vi "ET3500 - Write Program.vi"(5 "Simulate":bool caption="Simulate ET3500", 8 "Error In":errorcluster, 9 "MCListBox FHS Setup":refnum<vi>, 10 "WPS Details Setup":T3={"WPS/Ref"="", "Rev"="", "Hold Temperature"="80", "WPS Details Temperature Units"="DegC", "Hold Time (HH:MM)"="01:00", "Inactive"=FALSE} caption="WPS Details", 11 "VISA resource name RS232":string="visa://192.168.1.50/ASRL1::INSTR") -> (0 "ET3500":errorcluster, 1 "Final Target Temperture":i32, 2 "Duplicate Index":bool, 3 "Valid":bool, 4 "ET3500 Segment Table":i32[][](array[numeric])=[[1, 50, 400, 1], [2, 30, 500, 1], [3, 15, 600, 1], [4, 0, 0, 3], [5, 0, 0, 0]], 6 "Seq-Seg Info":T1)   [LabVIEW 2013]
uses:
  Controls/Combo Box.ctl
  Controls/ET3500 Enum.ctl
  Controls/ET3500 Programmer Enum.ctl
  Controls/ET3500 Segment Enum.ctl
panel:
  in  "Rev2":string="MyWPS55" caption="Rev"
  in  "Extra WPS":string="MyWPS55" caption="WPS"
  out "Old":i32[][](array[numeric])=[[1, 30, 300, 1], [2, 70, 600, 1], [0, 0, 0, 3], [5, 50, 400, 1], [0, 0, 0, 0]]
  out "Segment.Holdback":i32[](array[numeric])
  in  "ProgramNumber":i32=33
  out "num of rows\n(including blank row)":i32=4
  out "Main Hold Time (min)":dbl=270.0
  in  "MCListBox FHS Setup":i32(listbox)=-1 caption="Furnance Heating Sequence"
  # "visa://192.168.1.50/ASRL1::INSTR"
  # "Extra Fields used in SETUP ONLY"
  # "Sequence#       Ramp Rate       Target Temp          Hold Time       SegType"
  # "0 - NA\n1 - Low\n2 - High"
  # "Seq Num        Ramp Rate       Target Temp            SegType"
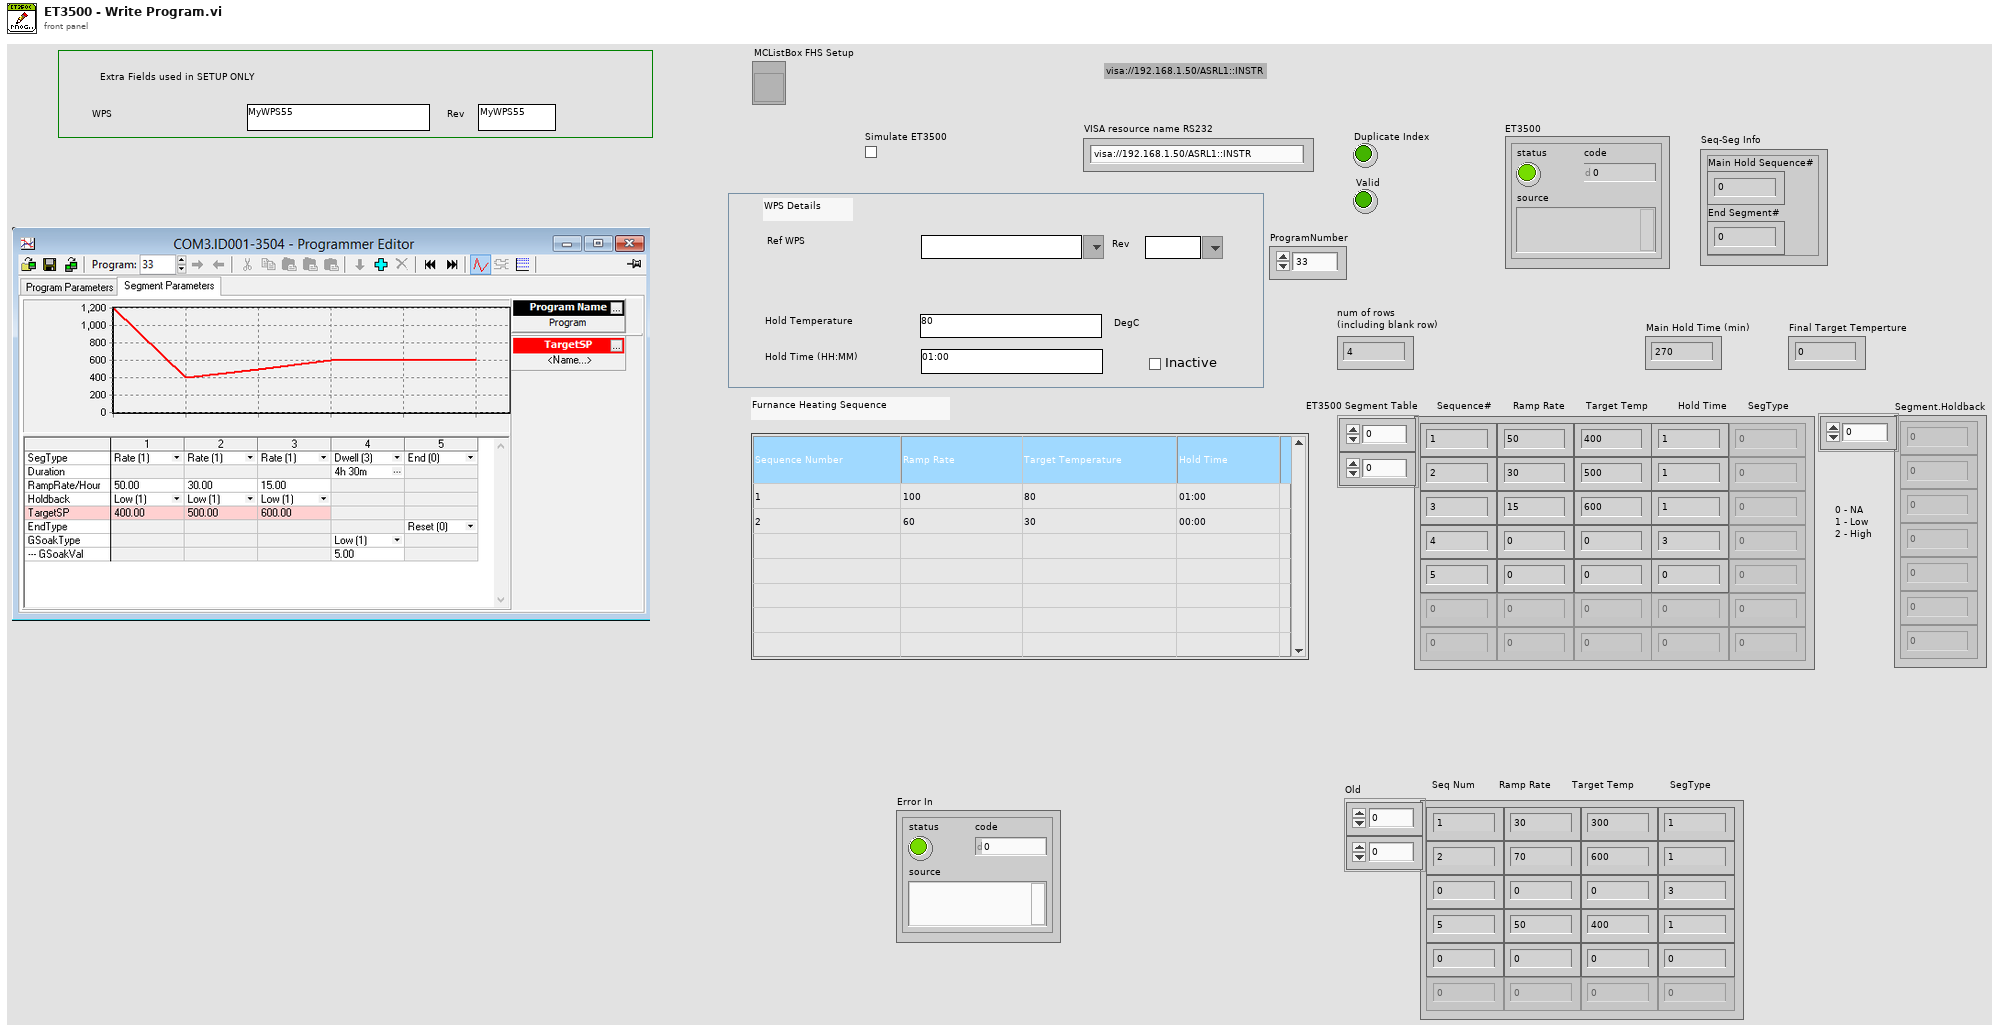
[diagram p1: front panel]
types:
  T1 = cluster{"Main Hold Sequence#":i32, "End Segment#":i32}
  T2 = typedef "Combo Box.ctl" = string
  T3 = cluster{"WPS/Ref":T2, "Rev":T2, "Hold Temperature":string, "WPS Details Temperature Units":string, "Hold Time (HH:MM)":string, "Inactive":bool}
  T4 = typedef "Enum - InteractiveMode-SubVIMode.ctl" = enum16{"Interactive", "subVI Mode"}
  T5 = typedef "ET3500 Enum.ctl" = enum16{"Programmer1", "Segment1", "Segment2", "Segment3", "Segment4", "Segment5", "Segment6", "Segment7", "Segment8", "Segment9", "Segment10", "Segment11", "Segment12", "Segment13", "Segment14", "Segment15", "Segment16"}
  T6 = typedef "ET3500 Programmer Enum.ctl" = u16
  T7 = typedef "ET3500 Segment Enum.ctl" = u16
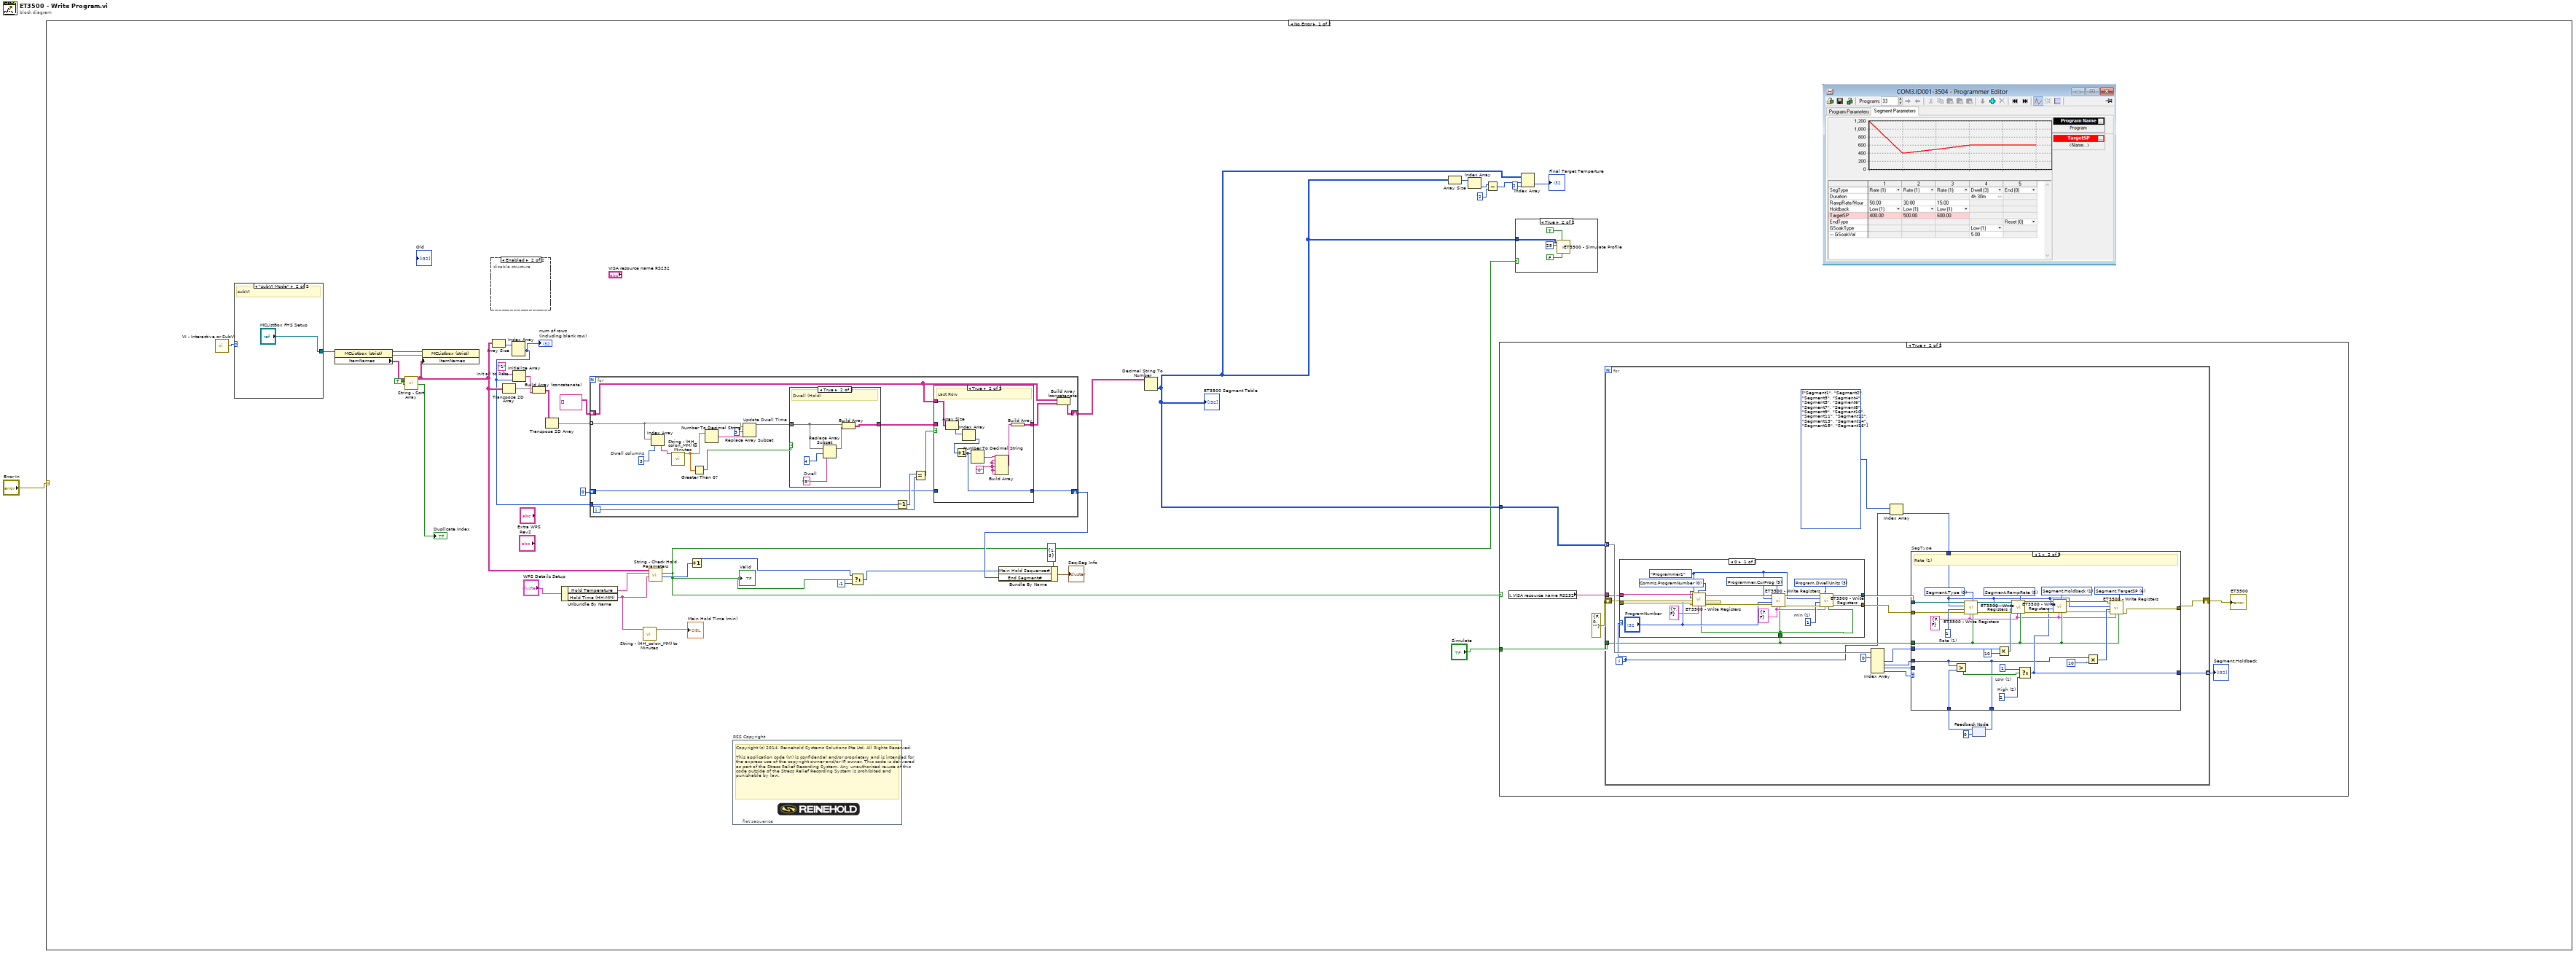
[diagram p0: block diagram]
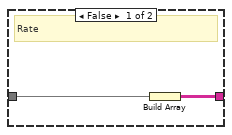
[diagram p3: hidden frame]
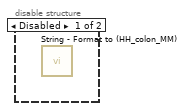
[diagram p4: hidden frame]
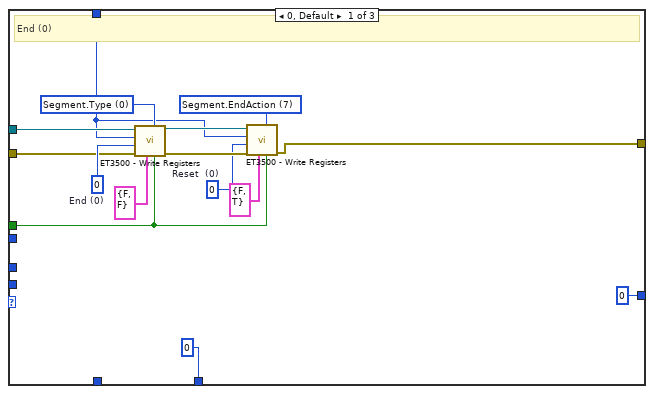
[diagram p8: hidden frame]
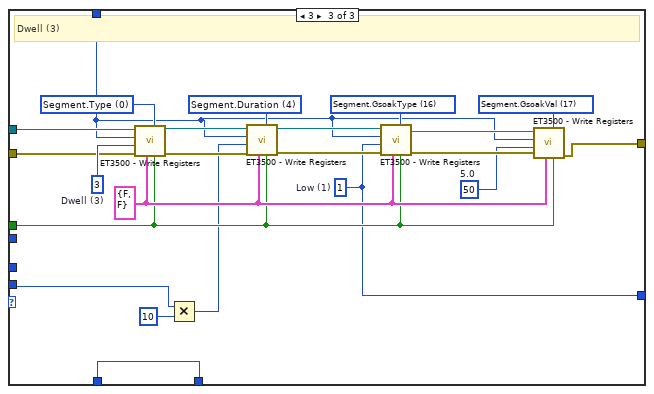
[diagram p9: hidden frame]
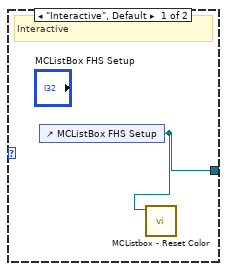
[diagram p10: hidden frame]
diagram:
  n1 = case shown="No Error" "Error In" {
    frame No Error {
      w12 = "1"  # Init all to Rate
      w11 = TRUE ("Check and Add Empty Row if Neccsary")
      n2 = call "VI - Interactive or SubVI.vi"() -> ("Mode"=w2:T4)  [unwired: 5 in]
      n3 = case shown="\"subVI Mode\"" w2 {
        tunnel: [w189 "MCListBox FHS Setup"] -> w34
        frame "Interactive", Default {
          # "Interactive"
          n4 = control-ref of="MCListBox FHS Setup"() -> (w189:refnum<vi>)
          n5 = call "MCListbox - Reset Color.vi"("MulticolumnListbox in"=w189) -> ()  [unwired: 10 in, 1 out]
        }
        frame "subVI Mode" {
          # "subVI"
        }
      }
      n6 = property class="MCListbox (strict)"(reference=w34) -> (reference out=w37:refnum<vi>, error out=w35:errorcluster, "ItemNames"=w36:string[][])  [unwired: 1 in]
      n7 = call "String - Sort Array.vi"("Force Running Numbers"=w11, "Check and Add Empty Row if Needed"=w11, "2D Array in"=w36) -> ("Duplicate Index"=→"Duplicate Index":bool, "2D Array out"=w19:string[][])  [unwired: 6 in, 1 out]
      n8 = property class="MCListbox (strict)"(reference=w37, error in=w35, "ItemNames"=w19) -> ()  [unwired: 2 out]
      n9 = disable-structure shown="Enabled" {
        frame Disabled {
          n10 = call "String - Format to (HH_colon_MM).vi"() -> ()  [unwired: 10 in, 2 out]
        }
        frame Enabled {
        }
      }
      n11 = Array Size(array=w19) -> (size(s)=w39:i32[])
      n12 = Transpose 2D Array(2D array=w19) -> (transposed array=w16:string[][])
      n13 = Index Array(array=w39) -> (element #1=w13:i32)  [unwired: 2 in, 1 out]
      "num of rows\n(including blank row)" <- w13
      n14 = Initialize Array(w12, w13) -> (w18:string[])
      n15 = Build Array (concatenate)(w16, w18) -> (w17:string[][])
      n16 = Transpose 2D Array(2D array=w17) -> (transposed array=w15:string[][])
      n17 = Unbundle By Name("WPS Details Setup") -> ("Hold Temperature"=w30:string, "Hold Time (HH:MM)"=w29:string)
      n18 = for {
        tunnel: w15 -> [w52] mode=indexing
        shift-right: [w53] -> w14
        shift-left: string[][] [] -> [w42]
        tunnel: w13 -> [w49]
        shift-right: [w41] -> w7
        shift-left: 0 -> [w40]
        i -> [w43]
        w54 = 3  # Dwell columns
        n19 = Index Array(array=w52, index=w54) -> (element=w57:string)
        n20 = call "String - (HH_colon_MM) to Minutes.vi"("Hold Time (HH:MM)"=w57) -> ("minutes"=w55:dbl)  [unwired: 10 in]
        n21 = Greater Than 0?(x=w55) -> (x > 0?=w56:bool)
        n22 = Number To Decimal String(number=w55) -> (decimal integer string=w51:string)  [unwired: 1 in]
        n23 = Replace Array Subset "Update Dwell Time"(array=w52, new element=w51, index=3) -> (w44:string[])
        n24 = case shown="True" w56 {
          tunnel: w44 -> [w68 w73]
          tunnel: [w69 w74] -> w46
          frame False {
            # "Rate"
            n25 = Build Array(w68) -> (w69:string[][])
          }
          frame True {
            w70 = "3"  # Dwell
            # "Dwell (Hold)"
            n26 = Replace Array Subset(array=w73, new element=w70, index=4) -> (w72:string[])
            n27 = Build Array(w73, w72) -> (w74:string[][])
          }
        }
        n28 = Decrement(x=w49) -> (x-1=w48:i32)
        n29 = Equal?(x=w48, y=w43) -> (x = y?=w47:bool)
        n30 = case shown="True" w47 {
          tunnel: w46 -> [w59 _]
          tunnel: [w59 w67] -> w45
          tunnel: w42 -> [_ w61]
          tunnel: [w58 w60] -> w41
          tunnel: w40 -> [w58 _]
          frame False {
          }
          frame True {
            w64 = "0" ("element")
            # "Last Row"
            n31 = Array Size(array=w61) -> (size(s)=w63:i32[])
            n32 = Index Array(array=w63) -> (element=w62:i32)  [unwired: 1 in]
            n33 = Increment(x=w62) -> (x+1=w60:i32)
            n34 = Number To Decimal String(number=w60) -> (decimal integer string=w66:string)  [unwired: 1 in]
            n35 = Build Array(w66, w64, w64, w64, w64, w64) -> (w65:string[])
            n36 = Build Array(w65) -> (w67:string[][])
          }
        }
        n37 = Build Array (concatenate)(w42, w45) -> (w53:string[][])
      }
      n38 = call "String - (HH_colon_MM) to Minutes.vi"("Hold Time (HH:MM)"=w29) -> ("minutes"=→"Main Hold Time (min)":dbl)  [unwired: 10 in]
      n39 = call "String - Check Hold Parameters.vi"("Master Data Hold Time (HH:MM)"=w29, "Master Data Hold Temperature"=w30, "2D Array in"=w19) -> ("index of Matched Hold Temperature"=w28:i32, "Found"=w6:bool)  [unwired: 6 in, 1 out]
      "Valid" <- w6
      n40 = Increment(x=w28) -> (x+1=w5:i32)
      n41 = flat-sequence "RSS Copyright" {
        frame #0 {
          # "Copyright (c) 2014, Reinehold Systems Solutions Pte Ltd. All Rights Reserved.\n\nThis application code (VI) is confidential and/or proprietary and is intended for the express use of the copyright owner and/or IP owner. This code is delivered as part of the Stress Relief Recording System. Any unauthorized re-use of this code outside of the Stress Relief Recording System is prohibited and punishable by law."
        }
      }
      n42 = Select(t=w5, s=w6, f=-1) -> (s? t:f=w3:i32)
      n43 = Bundle By Name(cluster=T1 {"Main Hold Sequence#"=1, "End Segment#"=5} ("Info"), "Main Hold Sequence#"=w3, "End Segment#"=w7) -> (→"Seq-Seg Info":T1)
      n44 = Decimal String To Number(string=w14) -> (number=w20:i32[][])  [unwired: 2 in, 1 out]
      "ET3500 Segment Table" <- w20
      n45 = Array Size(array=w20) -> (size(s)=w27:i32[])
      n46 = Index Array(array=w27) -> (element=w23:i32)  [unwired: 1 in]
      n47 = Subtract(x=w23, y=2 ("disabled index (col)")) -> (x-y=w26:i32)
      n48 = case shown="True" w6 {
        tunnel: w20 -> [_ w84]
        tunnel: "Simulate" -> [_ w80]
        frame False {
        }
        frame True {
          n49 = local read "VISA resource name RS232"() -> (w83:string)
          n50 = for {
            tunnel: w84 -> [w103] mode=indexing
            tunnel: w83 -> [w98]
            tunnel: w80 -> [w94]
            shift-right: [w99] -> w81
            shift-left: errorcluster {"status"=FALSE, "code"=0, "source"=""} ("error out") -> [w96]
            tunnel: [w90] -> w79 mode=indexing
            i -> [w92]
            w93 = T5[] [enum."Segment1", enum."Segment2", enum."Segment3", enum."Segment4", enum."Segment5", enum."Segment6", enum."Segment7", enum."Segment8", enum."Segment9", enum."Segment10", enum."Segment11", enum."Segment12", enum."Segment13", enum."Segment14", enum."Segment15", enum."Segment16"] items=["Programmer1", "Segment1", "Segment2", "Segment3", "Segment4", "Segment5", "Segment6", "Segment7", "Segment8", "Segment9", "Segment10", "Segment11", "Segment12", "Segment13", "Segment14", "Segment15", "Segment16"]
            n51 = case shown="0" w92 {
              tunnel: w98 -> [w116 w122]
              tunnel: [w112 w122] -> w97
              tunnel: w96 -> [w119 w121]
              tunnel: [w110 w121] -> w95
              tunnel: w94 -> [w104 _]
              frame 0 {
                w108 = 1  # min (1)
                w107 = T6 3 items=["Comms.ProgramNumber", "", "Program.RampUnits", "Program.DwellUnits", "", "", "", "", "", "Programmer.CurProg", "Programmer.CurSeg", "Programmer.ProgStatus", "", "", "", "", "", "Programmer.ProgTimeLeft", "Programmer.PVIn", "Programmer.SPIn", "", "Programmer.SegTimeLeft"] ("ET3500 Programmer Enum")
                w106 = T6 0 items=["Comms.ProgramNumber", "", "Program.RampUnits", "Program.DwellUnits", "", "", "", "", "", "Programmer.CurProg", "Programmer.CurSeg", "Programmer.ProgStatus", "", "", "", "", "", "Programmer.ProgTimeLeft", "Programmer.PVIn", "Programmer.SPIn", "", "Programmer.SegTimeLeft"] ("ET3500 Programmer Enum")
                w109 = ET3500_Enum."Programmer1" ("ET3500 Enum")
                w105 = cluster{"Init":bool, "Close":bool} {"Init"=FALSE, "Close"=FALSE} ("Option")
                w120 = T6 9 items=["Comms.ProgramNumber", "", "Program.RampUnits", "Program.DwellUnits", "", "", "", "", "", "Programmer.CurProg", "Programmer.CurSeg", "Programmer.ProgStatus", "", "", "", "", "", "Programmer.ProgTimeLeft", "Programmer.PVIn", "Programmer.SPIn", "", "Programmer.SegTimeLeft"] ("ET3500 Programmer Enum")
                n52 = call "ET3500 - Write Registers.vi"("Simulate"=w104, "Option"=cluster{"Init":bool, "Close":bool} {"Init"=TRUE, "Close"=FALSE}, "ET3500 Programmer Enum"=w106, "error in (no error)"=w119, "Process Variable  (0)"="ProgramNumber", "ET3500 Enum"=w109, "VISA resource name"=w116) -> ("error out"=w118:errorcluster, "VISA resource name out"=w117:refnum<visa-resource-name>)  [unwired: 3 in]
                n53 = call "ET3500 - Write Registers.vi"("Simulate"=w104, "Option"=w105, "ET3500 Programmer Enum"=w120, "error in (no error)"=w118, "Process Variable  (0)"="ProgramNumber", "ET3500 Enum"=w109, "VISA resource name"=w117) -> ("error out"=w111:errorcluster, "VISA resource name out"=w113:refnum<visa-resource-name>)  [unwired: 3 in]
                n54 = call "ET3500 - Write Registers.vi"("Simulate"=w104, "Option"=w105, "ET3500 Programmer Enum"=w107, "error in (no error)"=w111, "Process Variable  (0)"=w108, "ET3500 Enum"=w109, "VISA resource name"=w113) -> ("error out"=w110:errorcluster, "VISA resource name out"=w112:refnum<visa-resource-name>)  [unwired: 3 in]
              }
              frame 1, Default {
              }
            }
            n55 = Index Array(array=w103, index #1=0 ("index")) -> (element #2=w101:i32, element #3=w100:i32, element #4=w85:i32, element #5=w86:i32)  [unwired: 4 in, 1 out]
            n56 = Index Array(array=w93, index=w92) -> (element=w91:T5)
            n57 = feedback #1(0 ("String")) -> (w87:i32)
            n58 = case "SegType" shown="1" w86 {
              tunnel: w101 -> [_ w158 _]
              tunnel: w97 -> [w137 w165 w188]
              tunnel: w94 -> [w134 w148 w177]
              tunnel: w91 -> [w131 w154 w173]
              tunnel: w100 -> [_ w139 _]
              tunnel: [w127 w147 w171] -> w99
              tunnel: w95 -> [w126 w146 w182]
              tunnel: w85 -> [_ _ w166]
              tunnel: [0 ("Low (1)") w140 w168] -> w90
              tunnel: [0 ("String") w139 w167] -> w88
              tunnel: w87 -> [_ w138 w167]
              frame 0, Default {
                w129 = 0  # Reset  (0)
                w130 = T7 7 items=["Segment.Type", "Segment.Holdback", "", "", "Segment.Duration", "Segment.RampRate", "Segment.TargetSP", "Segment.EndAction", "", "", "", "", "", "", "", "", "Segment.GsoakType", "Segment.GsoakVal"] ("ET3500 Segment Enum")
                w136 = T7 0 items=["Segment.Type", "Segment.Holdback", "", "", "Segment.Duration", "Segment.RampRate", "Segment.TargetSP", "Segment.EndAction", "", "", "", "", "", "", "", "", "Segment.GsoakType", "Segment.GsoakVal"] ("ET3500 Segment Enum")
                w135 = 0  # End (0)
                # "End (0)"
                n59 = call "ET3500 - Write Registers.vi"("Simulate"=w134, "ET3500 Segment Enum"=w136, "Option"=cluster{"Init":bool, "Close":bool} {"Init"=FALSE, "Close"=FALSE}, "error in (no error)"=w126, "Process Variable  (0)"=w135, "ET3500 Enum"=w131, "VISA resource name"=w137) -> ("error out"=w133:errorcluster, "VISA resource name out"=w132:refnum<visa-resource-name>)  [unwired: 3 in]
                n60 = call "ET3500 - Write Registers.vi"("Simulate"=w134, "ET3500 Segment Enum"=w130, "Option"=cluster{"Init":bool, "Close":bool} {"Init"=FALSE, "Close"=TRUE}, "error in (no error)"=w133, "Process Variable  (0)"=w129, "ET3500 Enum"=w131, "VISA resource name"=w132) -> ("error out"=w127:errorcluster)  [unwired: 3 in, 1 out]
              }
              frame 1 {
                w141 = 2  # High (2)
                w142 = 1  # Low (1)
                w153 = T7 6 items=["Segment.Type", "Segment.Holdback", "", "", "Segment.Duration", "Segment.RampRate", "Segment.TargetSP", "Segment.EndAction", "", "", "", "", "", "", "", "", "Segment.GsoakType", "Segment.GsoakVal"] ("ET3500 Segment Enum")
                w145 = cluster{"Init":bool, "Close":bool} {"Init"=FALSE, "Close"=FALSE} ("Option")
                w155 = T7 1 items=["Segment.Type", "Segment.Holdback", "", "", "Segment.Duration", "Segment.RampRate", "Segment.TargetSP", "Segment.EndAction", "", "", "", "", "", "", "", "", "Segment.GsoakType", "Segment.GsoakVal"] ("ET3500 Segment Enum")
                w160 = T7 5 items=["Segment.Type", "Segment.Holdback", "", "", "Segment.Duration", "Segment.RampRate", "Segment.TargetSP", "Segment.EndAction", "", "", "", "", "", "", "", "", "Segment.GsoakType", "Segment.GsoakVal"] ("ET3500 Segment Enum")
                w164 = T7 0 items=["Segment.Type", "Segment.Holdback", "", "", "Segment.Duration", "Segment.RampRate", "Segment.TargetSP", "Segment.EndAction", "", "", "", "", "", "", "", "", "Segment.GsoakType", "Segment.GsoakVal"] ("ET3500 Segment Enum")
                w163 = 1  # Rate (1)
                # "Rate (1)"
                n61 = Greater?(x=w139, y=w138) -> (0:w143:bool)
                n62 = call "ET3500 - Write Registers.vi"("Simulate"=w148, "ET3500 Segment Enum"=w164, "Option"=w145, "error in (no error)"=w146, "Process Variable  (0)"=w163, "ET3500 Enum"=w154, "VISA resource name"=w165) -> ("error out"=w162:errorcluster, "VISA resource name out"=w161:refnum<visa-resource-name>)  [unwired: 3 in]
                n63 = Multiply(x=w158, y=10) -> (x*y=w157:i32)
                n64 = call "ET3500 - Write Registers.vi"("Simulate"=w148, "ET3500 Segment Enum"=w160, "Option"=w145, "error in (no error)"=w162, "Process Variable  (0)"=w157, "ET3500 Enum"=w154, "VISA resource name"=w161) -> ("error out"=w150:errorcluster, "VISA resource name out"=w156:refnum<visa-resource-name>)  [unwired: 3 in]
                n65 = Select(t=w142, s=w143, f=w141) -> (s? t:f=w140:i32)
                n66 = call "ET3500 - Write Registers.vi"("Simulate"=w148, "ET3500 Segment Enum"=w155, "Option"=w145, "error in (no error)"=w150, "Process Variable  (0)"=w140, "ET3500 Enum"=w154, "VISA resource name"=w156) -> ("error out"=w149:errorcluster, "VISA resource name out"=w144:refnum<visa-resource-name>)  [unwired: 3 in]
                n67 = Multiply(x=w139, y=10) -> (x*y=w151:i32)
                n68 = call "ET3500 - Write Registers.vi"("Simulate"=w148, "ET3500 Segment Enum"=w153, "Option"=w145, "error in (no error)"=w149, "Process Variable  (0)"=w151, "ET3500 Enum"=w154, "VISA resource name"=w144) -> ("error out"=w147:errorcluster)  [unwired: 3 in, 1 out]
              }
              frame 3 {
                w172 = T7 17 items=["Segment.Type", "Segment.Holdback", "", "", "Segment.Duration", "Segment.RampRate", "Segment.TargetSP", "Segment.EndAction", "", "", "", "", "", "", "", "", "Segment.GsoakType", "Segment.GsoakVal"] ("ET3500 Segment Enum")
                w176 = 50  # 5.0
                w168 = 1  # Low (1)
                w180 = T7 16 items=["Segment.Type", "Segment.Holdback", "", "", "Segment.Duration", "Segment.RampRate", "Segment.TargetSP", "Segment.EndAction", "", "", "", "", "", "", "", "", "Segment.GsoakType", "Segment.GsoakVal"] ("ET3500 Segment Enum")
                w178 = cluster{"Init":bool, "Close":bool} {"Init"=FALSE, "Close"=FALSE} ("Option")
                w183 = T7 4 items=["Segment.Type", "Segment.Holdback", "", "", "Segment.Duration", "Segment.RampRate", "Segment.TargetSP", "Segment.EndAction", "", "", "", "", "", "", "", "", "Segment.GsoakType", "Segment.GsoakVal"] ("ET3500 Segment Enum")
                w187 = T7 0 items=["Segment.Type", "Segment.Holdback", "", "", "Segment.Duration", "Segment.RampRate", "Segment.TargetSP", "Segment.EndAction", "", "", "", "", "", "", "", "", "Segment.GsoakType", "Segment.GsoakVal"] ("ET3500 Segment Enum")
                w186 = 3  # Dwell (3)
                # "Dwell (3)"
                n69 = call "ET3500 - Write Registers.vi"("Simulate"=w177, "ET3500 Segment Enum"=w187, "Option"=w178, "error in (no error)"=w182, "Process Variable  (0)"=w186, "ET3500 Enum"=w173, "VISA resource name"=w188) -> ("error out"=w185:errorcluster, "VISA resource name out"=w184:refnum<visa-resource-name>)  [unwired: 3 in]
                n70 = Multiply(x=w166, y=10) -> (x*y=w169:i32)
                n71 = call "ET3500 - Write Registers.vi"("Simulate"=w177, "ET3500 Segment Enum"=w183, "Option"=w178, "error in (no error)"=w185, "Process Variable  (0)"=w169, "ET3500 Enum"=w173, "VISA resource name"=w184) -> ("error out"=w181:errorcluster, "VISA resource name out"=w174:refnum<visa-resource-name>)  [unwired: 3 in]
                n72 = call "ET3500 - Write Registers.vi"("Simulate"=w177, "ET3500 Segment Enum"=w180, "Option"=w178, "error in (no error)"=w181, "Process Variable  (0)"=w168, "ET3500 Enum"=w173, "VISA resource name"=w174) -> ("error out"=w179:errorcluster, "VISA resource name out"=w175:refnum<visa-resource-name>)  [unwired: 3 in]
                n73 = call "ET3500 - Write Registers.vi"("Simulate"=w177, "ET3500 Segment Enum"=w172, "Option"=w178, "error in (no error)"=w179, "Process Variable  (0)"=w176, "ET3500 Enum"=w173, "VISA resource name"=w175) -> ("error out"=w171:errorcluster)  [unwired: 3 in, 1 out]
              }
            }
            n74 = feedback-in #1(w88) -> ()
          }
          "ET3500" <- w81
          "Segment.Holdback" <- w79
        }
      }
      n75 = case shown="True" w6 {
        tunnel: w20 -> [_ w78]
        frame False {
        }
        frame True {
          n76 = call "ET3500 - Simulate Profile.vi"("Popup"=FALSE ("subVI"), "Set (T) / Get (F)"=TRUE, "Start Temp"=25, "Final Segments"=w78) -> ()  [unwired: 3 in, 5 out]
        }
      }
      n77 = Index Array(array=w20, index (row)=w26, index (col)=2 ("disabled index (col)")) -> (element=→"Final Target Temperture":i32)
    }
    frame Error {
    }
  }
